vi "canopen_monitor.vi"   [LabVIEW 2011]
uses:
  canopen_dll_master.dll
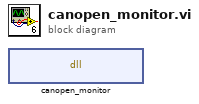
[diagram p0: block diagram]
diagram:
  n1 = dll-call lib="canopen_dll_master.dll" fn="canopen_monitor"() -> ()  [unwired: 4 in, 2 out]
